vi "macro_Pose2d_XYAngleRad.vi"   [LabVIEW 2019, in "Trajectory_Library.lvlib"]
uses:
  Trajectory_Library.lvlib
  Rotation2d_CreateAngle.vi
  Translation2d_Create.vi
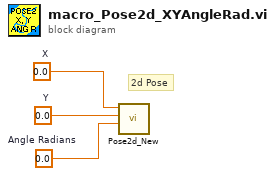
[diagram p0: block diagram]
diagram:
  w2 = 0.0  # X
  w3 = 0.0  # Y
  w1 = 0.0  # Angle Radians
  # "2d Pose"
  n1 = call "Pose2d_New.vi"("Heading"=w1, "Y"=w3, "X"=w2) -> ()  [unwired: 8 in, 1 out]
